vi "setScriptInfo.vi"(8 "error in (no error)":errorcluster, 10 "Script info":string, 11 "DataPointScript.lvclass in":refnum<class "DataPointScript.lvclass">) -> (0 "error out":errorcluster, 3 "DataPointScript.lvclass out":refnum<class "DataPointScript.lvclass">)   [LabVIEW 2009, in "Tools.lvlib" / "Scripting.lvlib" / "DataPointScript.lvclass"]
uses:
  DataPointScript.lvclass
  DataPointScript.lvclass/DataPointScript.ctl
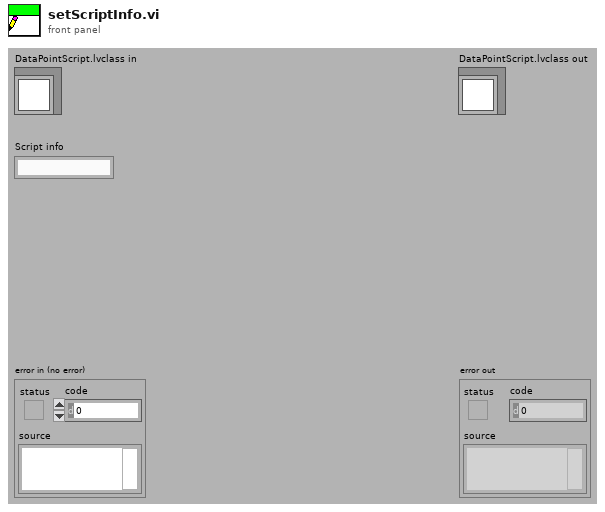
[diagram p1: front panel]
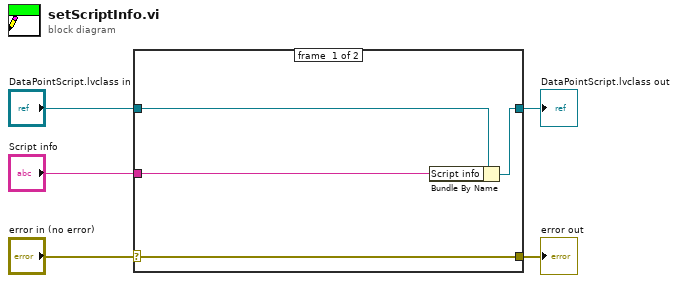
[diagram p0: block diagram]
diagram:
  n1 = case shown="No Error" "error in (no error)" {
    selector: "error in (no error)" -> [w9 w10]
    tunnel: [w9 w10] -> w4
    tunnel: [w7 w11] -> w2
    tunnel: "DataPointScript.lvclass in" -> [w8 w11]
    tunnel: "Script info" -> [w6 _]
    frame #0 {
      n2 = Bundle By Name(cluster=w8, "Script info"=w6) -> (w7:refnum<class "DataPointScript.lvclass">)
    }
    frame #1 {
    }
  }
  "error out" <- w4
  "DataPointScript.lvclass out" <- w2
